vi "find_centroid.vi"(5 "Selection and Groups":T3[](array[typedef]), 8 "Spots":T1[](array[typedef]) {"Amplitude Correction" step=0.1; "Line Trapping"."Phase Gradient" step=0.05; "Line Trapping"."Vector"."x" step=1e-06 format="%#_6p"; "Line Trapping"."Vector"."y" step=1e-06 format="%#_6p"; "Line Trapping"."Vector"."z" step=1e-06 format="%#_6p"; "NA Position"."r" step=1e-06; "NA Position"."y" step=1e-06; "NA Position"."x" step=1e-06; "Position"."z" step=1e-06; "Position"."y" step=1e-06; "Position"."x" step=1e-06; "Phase" step=0.7753; "Intensity" step=0.1}) -> (0 "centroid (2d)":cluster{"x":dbl, "y":dbl}, 1 "Mean Values":T1={"Position"={"x"=0.0, "y"=0.0, "z"=0.0}, "Intensity"=1.0, "Vortex Charge"=1, "Phase"=1.0, "NA Position"={"x"=0.0, "y"=0.0, "r"=1.0}, "Line Trapping"={"Vector"={"x"=0.0, "y"=0.0, "z"=0.0}, "Phase Gradient"=0.0}, "Amplitude Correction"=0.0} {"Amplitude Correction" step=0.1; "Line Trapping"."Phase Gradient" step=0.05; "Line Trapping"."Vector"."x" step=1e-06 format="%#_6p"; "Line Trapping"."Vector"."y" step=1e-06 format="%#_6p"; "Line Trapping"."Vector"."z" step=1e-06 format="%#_6p"; "NA Position"."r" step=1e-06; "NA Position"."y" step=1e-06; "NA Position"."x" step=1e-06; "Position"."z" step=1e-06; "Position"."y" step=1e-06; "Position"."x" step=1e-06; "Phase" step=0.7753; "Intensity" step=0.1}, 2 "size":cluster{"x":dbl, "y":dbl, "z":dbl}, 3 "centroid":cluster{"x":dbl, "y":dbl, "z":dbl}, 4 "# selected":i16)   [LabVIEW 2010]
doc: "Finds the mean value of the selected spots (or all spots if selection is not wired). It also extracts the position and x-y position for convenience."
uses:
  spot.ctl
  line_trapping.ctl
  selection_element.ctl
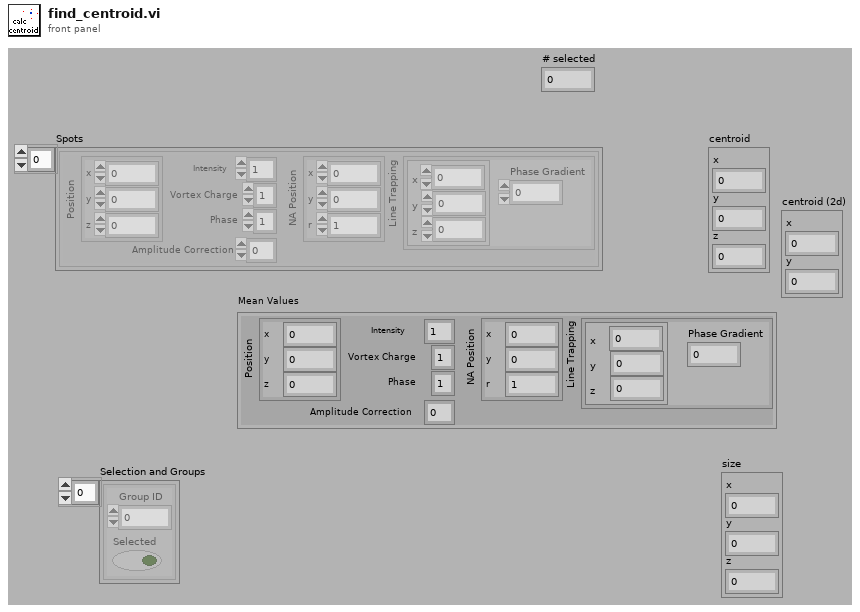
[diagram p1: front panel]
types:
  T1 = typedef "spot.ctl" = cluster{"Position":cluster{"x":dbl, "y":dbl, "z":dbl}, "Intensity":dbl, "Vortex Charge":i8, "Phase":dbl, "NA Position":cluster{"x":dbl, "y":dbl, "r":dbl}, "Line Trapping":T2, "Amplitude Correction":dbl}
  T2 = typedef "line_trapping.ctl" = cluster{"Vector":cluster{"x":dbl, "y":dbl, "z":dbl}, "Phase Gradient":dbl}
  T3 = typedef "selection_element.ctl" = cluster{"Group ID":i32, "Selected":bool}
  T4 = cluster{"Position":cluster{"x":dbl, "y":dbl, "z":dbl}, "Intensity":dbl, "Vortex Charge":i16, "Phase":dbl, "NA Position":cluster{"x":dbl, "y":dbl, "r":dbl}, "Line Trapping":T2, "Amplitude Correction":dbl}
  T5 = cluster{"Position":cluster{"x":dbl, "y":dbl, "z":dbl}, "Intensity":dbl, "Vortex Charge":dbl, "Phase":dbl, "NA Position":cluster{"x":dbl, "y":dbl, "r":dbl}, "Line Trapping":T2, "Amplitude Correction":dbl}
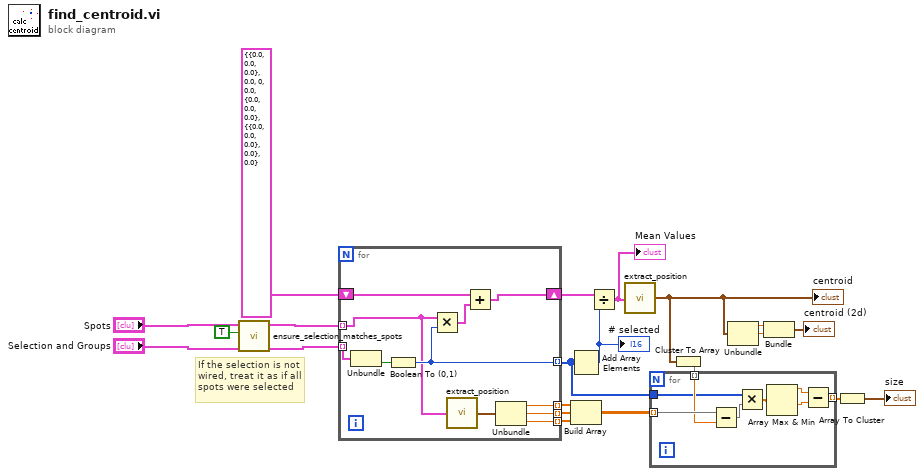
[diagram p0: block diagram]
diagram:
  # "If the selection is not wired, treat it as if all spots were selected"
  n1 = call "ensure_selection_matches_spots.vi"("Selection and Groups in"="Selection and Groups", "Select All (default: no)"=TRUE ("Select All (default: true)"), "Spots"="Spots") -> ("Selection and Groups out"=w14:T3[])  [unwired: 3 in, 1 out]
  n2 = for {
    tunnel: "Spots" -> [w25] mode=indexing
    tunnel: w14 -> [w31] mode=indexing
    shift-right: [w28] -> w19
    shift-left: T1 {"Position"={"x"=0.0, "y"=0.0, "z"=0.0}, "Intensity"=0.0, "Vortex Charge"=0, "Phase"=0.0, "NA Position"={"x"=0.0, "y"=0.0, "r"=0.0}, "Line Trapping"={"Vector"={"x"=0.0, "y"=0.0, "z"=0.0}, "Phase Gradient"=0.0}, "Amplitude Correction"=0.0} ("Cluster") -> [w27]
    tunnel: [w26] -> w4 mode=indexing
    tunnel: [w23] -> w8 mode=indexing
    tunnel: [w22] -> w9 mode=indexing
    tunnel: [w21] -> w10 mode=indexing
    n3 = Unbundle(w31) -> ("Selected"=w30:bool)  [unwired: 1 out]
    n4 = Boolean To (0,1)(Boolean=w30) -> (0, 1=w26:i16)
    n5 = Multiply(x=w25, y=w26) -> (x*y=w29:T4)
    n6 = call "extract_position.vi"("Spot"=w25) -> ("Position"=w24:cluster{"x":dbl, "y":dbl, "z":dbl})
    n7 = Add(x=w27, y=w29) -> (x+y=w28:T4)
    n8 = Unbundle(w24) -> ("x"=w23:dbl, "y"=w22:dbl, "z"=w21:dbl)
  }
  n9 = Add Array Elements(numeric array=w4) -> (sum=w20:i16)
  "# selected" <- w20
  n10 = Build Array(w8, w9, w10) -> (w6:dbl[][])
  n11 = Divide(x=w19, y=w20) -> (x/y=w12:T5)
  "Mean Values" <- w12
  n12 = call "extract_position.vi"("Spot"=w12) -> ("Position"=w7:cluster{"x":dbl, "y":dbl, "z":dbl})
  "centroid" <- w7
  n13 = Cluster To Array(cluster=w7) -> (array=w5:dbl[])
  n14 = for {
    tunnel: w6 -> [w39] mode=indexing
    tunnel: w5 -> [w38] mode=indexing
    tunnel: w4 -> [w36]
    tunnel: [w32] -> w3 mode=indexing
    n15 = Subtract(x=w39, y=w38) -> (x-y=w37:dbl[])
    n16 = Multiply(x=w36, y=w37) -> (x*y=w35:dbl[])
    n17 = Array Max & Min(array=w35) -> (max value=w33:dbl, min value=w34:dbl)  [unwired: 2 out]
    n18 = Subtract(x=w33, y=w34) -> (x-y=w32:dbl)
  }
  n19 = Unbundle(w7) -> ("x"=w18:dbl, "y"=w17:dbl)  [unwired: 1 out]
  n20 = Bundle("x"=w18, "y"=w17) -> (→"centroid (2d)":cluster{"x":dbl, "y":dbl})  [unwired: 1 out]
  n21 = Array To Cluster(array=w3) -> (cluster=→"size":cluster{"[0]":dbl, "[1]":dbl, "[2]":dbl})
